vi "Solve1.vi"(8 "Error In":errorcluster, 11 "object in":refnum<class "2022_5.lvclass">) -> (0 "Error Out":errorcluster, 2 "Result":u64, 3 "object out":refnum<class "2022_5.lvclass">)   [LabVIEW 2020, in "2022_5.lvclass"]
uses:
  2022_5.lvclass
  2022_5.lvclass/2022_5.ctl
panel:
  out "TopCrates":string
  out "Move":cluster{"Qty":i32, "From":i32, "To":i32}
  out "StacksOut":string[][](array[string])
  out "StacksIn":string[][](array[string])
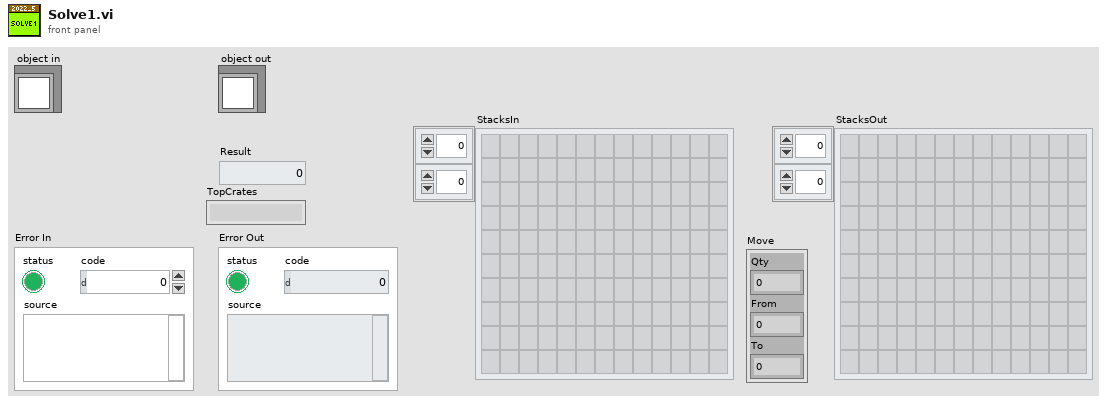
[diagram p1: front panel]
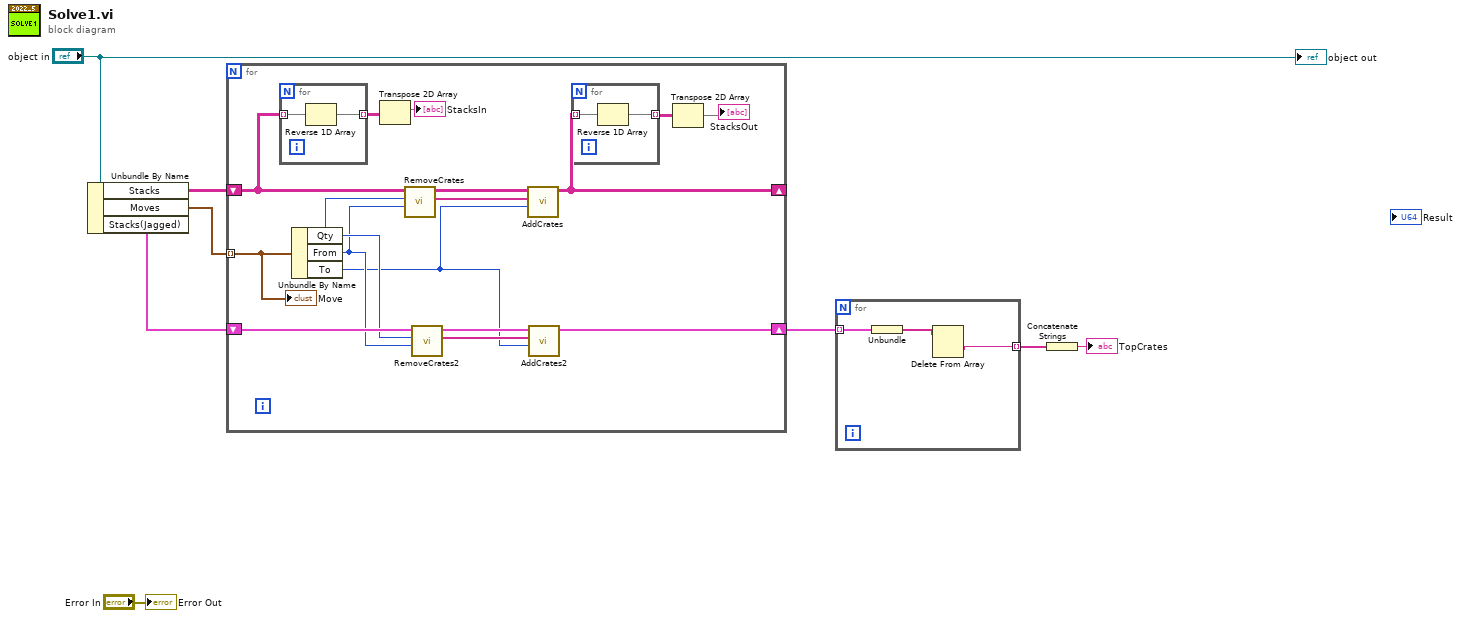
[diagram p0: block diagram]
diagram:
  n1 = Unbundle By Name("object in") -> ("Stacks"=w6:string[][], "Moves"=w5:cluster{"Qty":i32, "From":i32, "To":i32}[], "Stacks(Jagged)"=w4:cluster{"Crates":string[]}[])
  n2 = for {
    shift-right: [w18] -> _
    shift-left: w6 -> [w20]
    tunnel: w5 -> [w21] mode=indexing
    shift-right: [w11] -> w3
    shift-left: w4 -> [w15]
    n3 = for {
      tunnel: w20 -> [w28] mode=indexing
      tunnel: [w27] -> w19 mode=indexing
      n4 = Reverse 1D Array(array=w28) -> (reversed array=w27:string[])
    }
    n5 = Unbundle By Name(w21) -> ("Qty"=w14:i32, "From"=w13:i32, "To"=w9:i32)
    n6 = Transpose 2D Array(2D array=w19) -> (transposed array=→"StacksIn":string[][])
    n7 = call "RemoveCrates.vi"("From"=w13, "Qty"=w14, "StacksIn"=w20) -> ("CratesRemoved"=w23:string[], "StacksOut"=w24:string[][])  [unwired: 7 in]
    n8 = call "RemoveCrates2.vi"("From"=w13, "Qty"=w14, "StacksIn"=w15) -> ("CratesRemoved"=w10:string[], "StacksOut"=w12:cluster{"Crates":string[]}[])  [unwired: 7 in]
    n9 = call "AddCrates.vi"("To"=w9, "CratesToAdd"=w23, "StacksIn"=w24) -> ("StacksOut"=w18:string[][])  [unwired: 8 in]
    n10 = call "AddCrates2.vi"("To"=w9, "CratesToAdd"=w10, "StacksIn"=w12) -> ("StacksOut"=w11:cluster{"Crates":string[]}[])  [unwired: 8 in]
    n11 = for {
      tunnel: w18 -> [w26] mode=indexing
      tunnel: [w25] -> w17 mode=indexing
      n12 = Reverse 1D Array(array=w26) -> (reversed array=w25:string[])
    }
    n13 = Transpose 2D Array(2D array=w17) -> (transposed array=→"StacksOut":string[][])
    "Move" <- w21
  }
  n14 = for {
    tunnel: w3 -> [w31] mode=indexing
    tunnel: [w29] -> w2 mode=indexing
    n15 = Unbundle(w31) -> ("Crates"=w30:string[])
    n16 = Delete From Array(array=w30) -> (deleted portion=w29:string)  [unwired: 2 in, 1 out]
  }
  n17 = Concatenate Strings(w2) -> (→"TopCrates":string)
  "Error Out" <- "Error In"
  "object out" <- "object in"
